vi "Read Diode.vi"(8 "error in (no error)":errorcluster, 11 "Meter In":refnum<class "Meter.lvclass">) -> (0 "error out":errorcluster, 2 "Diode Voltage":dbl, 3 "Meter Out":refnum<class "Meter.lvclass">)   [LabVIEW 2019, in "Meter.lvclass"]
uses:
  Meter.lvclass
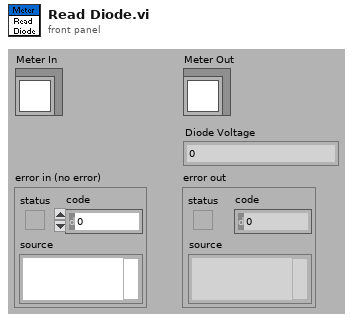
[diagram p1: front panel]
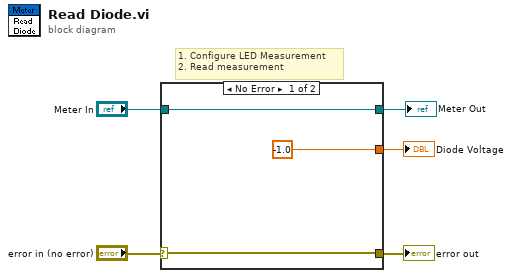
[diagram p0: block diagram]
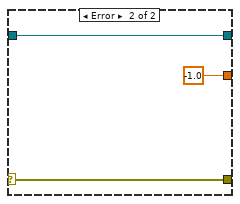
[diagram p2: hidden frame]
diagram:
  # "1. Configure LED Measurement\n2. Read measurement"
  n1 = case shown="No Error" "error in (no error)" {
    selector: "error in (no error)" -> [w6 w9]
    tunnel: [w6 w9] -> w4
    tunnel: [w8 w11] -> w1
    tunnel: "Meter In" -> [w8 w11]
    tunnel: [-1.0 -1.0] -> w3
    frame No Error {
    }
    frame Error {
    }
  }
  "error out" <- w4
  "Diode Voltage" <- w3
  "Meter Out" <- w1
